vi "EPR measure with dot tracking.vi"() -> ()   [LabVIEW 2011]
uses:
  <vilib>/DAQmx/write.llb/DAQmx Write (Digital Bool 1Line 1Point).vi
  <vilib>/DAQmx/create/channels.llb/DAQmx Create Channel (DO-Digital Output).vi
  <vilib>/DAQmx/miscellaneous.llb/DAQmx Fill In Error Info.vi
panel:
  in  "file path":path
  in  "N loops":i32=-1
  in  "Tracking Interval":dbl
  in  "Total Time":dbl
  out "Cross Section Y":dbl[](graph)
  out "Cross Section X":dbl[](graph)
  in  "Z-track?":bool=TRUE
  out "Gave up?":bool
  out "Z Position":dbl
  out "Y Position":dbl
  out "X Position":dbl
  in  "Z Pos":dbl=52.1
  in  "RS232 settings":cluster{"Portnumber":i32, "Baudrate":u16}={"Portnumber"=12, "Baudrate"=5} {"Portnumber" items=["COM1", "COM2", "COM3", "COM4", "COM5", "COM6", "COM7", "COM8", "COM9", "COM10", "COM11", "COM12", "COM13", "COM14", "COM15", "COM16", "COM17", "COM18", "COM19", "COM20", "COM21", "COM22", "COM23", "COM24", "COM25", "COM26", "COM27", "COM28", "COM29", "COM30"]; "Baudrate" items=["9600", "14400", "19200", "38400", "57600", "115200"]}
  in  "Y Parameters":T1={"Number of Y Steps"=200, "Max Y (V)"=2.0, "Min Y (V)"=-2.0}
  in  "X Parameters":T2={"Number of X Steps"=200, "Max X (V)"=2.0, "Min X (V)"=-2.0}
  in  "X Pos":dbl=192.0
  in  "Y pos":dbl=35.0
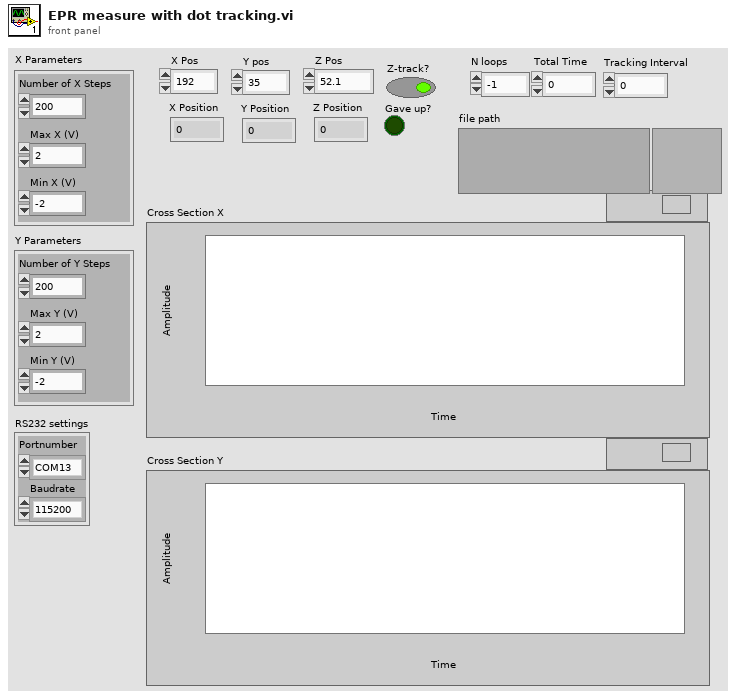
[diagram p1: front panel]
types:
  T1 = cluster{"Number of Y Steps":i32, "Max Y (V)":dbl, "Min Y (V)":dbl}
  T2 = cluster{"Number of X Steps":i32, "Max X (V)":dbl, "Min X (V)":dbl}
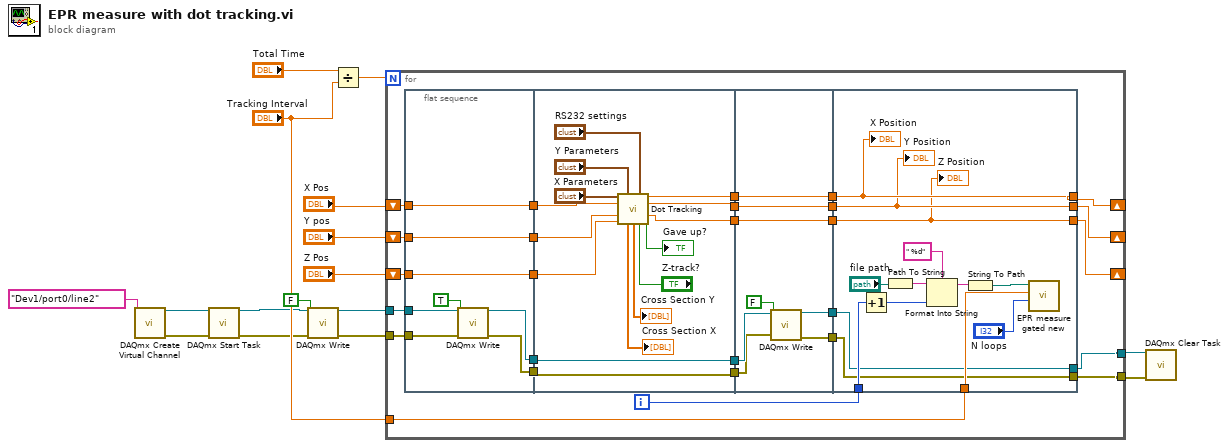
[diagram p0: block diagram]
diagram:
  n1 = call-poly <vilib>:"DAQmx Create Virtual Channel.vi"("lines"=tag "Dev1/port0/line2") -> ("task out"=w9:refnum<k21>, "error out"=w6:errorcluster)  [unwired: 13 in]
  n2 = call <vilib>:"DAQmx Start Task.vi"("task/channels in"=w9, "error in"=w6) -> ("task out"=w4:refnum<k21>, "error out"=w3:errorcluster)  [unwired: 12 in]
  n3 = call-poly <vilib>:"DAQmx Write.vi"("task/channels in"=w4, "data"=FALSE, "error in"=w3) -> ("task out"=w1:refnum<k21>, "error out"=w2:errorcluster)  [unwired: 10 in, 1 out]
  n4 = Divide(x="Total Time", y="Tracking Interval") -> (x/y=w13:dbl)
  n5 = for {
    N: w13 -> [_]
    shift-right: [w17] -> _
    shift-left: "X Pos" -> [w43]
    shift-right: [w18] -> _
    shift-left: "Y pos" -> [w42]
    shift-right: [w19] -> _
    shift-left: "Z Pos" -> [w41]
    tunnel: "Tracking Interval" -> [w40]
    tunnel: w1 -> [w35]
    tunnel: w2 -> [w34]
    tunnel: [w23] -> w8
    tunnel: [w20] -> w7
    i -> [w39]
    n6 = flat-sequence {
      tunnel: w41 -> [w49]
      tunnel: w42 -> [w50]
      tunnel: w43 -> [w51]
      tunnel: [w51] -> w38
      tunnel: [w50] -> w37
      tunnel: [w49] -> w36
      tunnel: w35 -> [w48]
      tunnel: w34 -> [w47]
      tunnel: [w45] -> w26
      tunnel: [w44] -> w24
      tunnel: [w59] -> w33
      tunnel: [w58] -> w31
      tunnel: [w57] -> w29
      tunnel: w38 -> [w63]
      tunnel: w37 -> [w62]
      tunnel: w36 -> [w61]
      tunnel: [w53] -> w27
      tunnel: w26 -> [w53]
      tunnel: [w52] -> w25
      tunnel: w24 -> [w52]
      tunnel: w33 -> [w74]
      tunnel: [w74] -> w32
      tunnel: w31 -> [w73]
      tunnel: [w73] -> w30
      tunnel: w29 -> [w72]
      tunnel: [w72] -> w28
      tunnel: w27 -> [w71]
      tunnel: w25 -> [w70]
      tunnel: [w68] -> w22
      tunnel: [w67] -> w21
      tunnel: w32 -> [w88]
      tunnel: [w87] -> w18
      tunnel: w30 -> [w87]
      tunnel: [w86] -> w19
      tunnel: w28 -> [w86]
      tunnel: [w88] -> w17
      tunnel: w40 -> [w84]
      tunnel: w39 -> [w82]
      tunnel: [w77] -> w23
      tunnel: w22 -> [w77]
      tunnel: w21 -> [w76]
      tunnel: [w76] -> w20
      frame #0 {
        n7 = call-poly <vilib>:"DAQmx Write.vi"("task/channels in"=w48, "data"=TRUE, "error in"=w47) -> ("task out"=w45:refnum<k21>, "error out"=w44:errorcluster)  [unwired: 10 in, 1 out]
      }
      frame #1 {
        n8 = call "Dot Tracking.vi"("X Parameters"="X Parameters", "Y Parameters"="Y Parameters", "RS232 settings"="RS232 settings", "X Pos"=w63, "Y pos"=w62, "Z Pos"=w61, "Z-track?"="Z-track?") -> ("X Position"=w59:dbl, "Y Position"=w58:dbl, "Z Position"=w57:dbl, "Cross Section X"=→"Cross Section X":dbl[], "Cross Section Y"=→"Cross Section Y":dbl[], "Gave up?"=→"Gave up?":bool)  [unwired: 3 in]
      }
      frame #2 {
        n9 = call-poly <vilib>:"DAQmx Write.vi"("task/channels in"=w71, "data"=FALSE, "error in"=w70) -> ("task out"=w68:refnum<k21>, "error out"=w67:errorcluster)  [unwired: 10 in, 1 out]
      }
      frame #3 {
        n10 = Increment(x=w82) -> (x+1=w75:i32)
        n11 = Path To String(path="file path") -> (string=w80:string)
        n12 = Format Into String(format string=" %d", initial string=w80, w75) -> (resulting string=w79:string)  [unwired: 1 in, 1 out]
        n13 = String To Path(string=w79) -> (path=w78:path)
        n14 = call "EPR measure gated new.vi"("N loops"="N loops", "Measurement Interval"=w84, "file path (dialog if empty)"=w78) -> ()  [unwired: 9 in]
        "X Position" <- w88
        "Y Position" <- w87
        "Z Position" <- w86
      }
    }
  }
  n15 = call <vilib>:"DAQmx Clear Task.vi"("task in"=w8, "error in"=w7) -> ()  [unwired: 13 in, 1 out]
